vi "Picture to 2-D Color Array.vi"(8 "에러 입력":errorcluster, 10 "입력 클러스터":cluster{"Width":u32, "Height":u32}, 11 "그림":picture) -> (0 "에러 출력":errorcluster, 3 "색 배열":cluster{"Red":u8, "Green":u8, "Blue":u8}[][](array[cluster]))   [LabVIEW 2010]
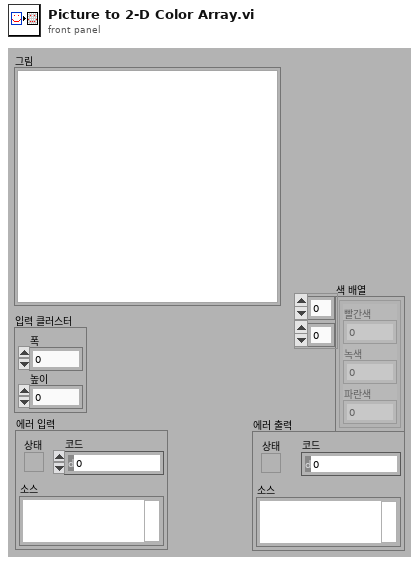
[diagram p1: front panel]
types:
  T1 = cluster{"left":i16, "top":i16, "right":i16, "bottom":i16}
  T2 = typedef "imagedata.ctl" = cluster{"image type":i32, "image depth":i32, "image":u8[], "mask":u8[], "colors":u32[], "Rectangle":cluster{"left":i16, "top":i16, "right":i16, "bottom":i16}}
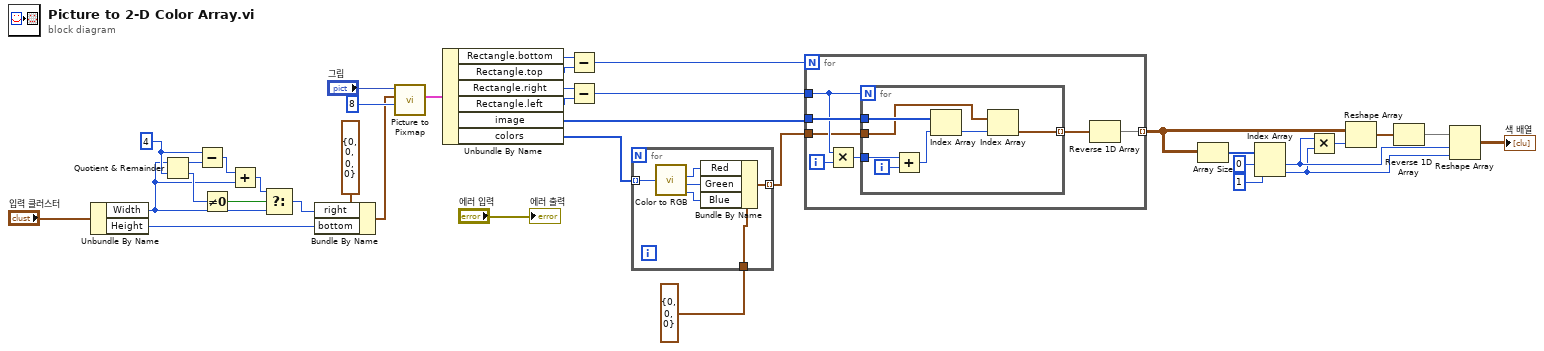
[diagram p0: block diagram]
diagram:
  w21 = 4
  n1 = Unbundle By Name("입력 클러스터") -> ("Width"=w4:u32, "Height"=w25:u32)
  n2 = Quotient & Remainder(x=w4, y=w21) -> (x-y*floor(x/y)=w20:u32, floor(x/y)=w19:u32)
  n3 = Subtract(x=w21, y=w20) -> (x-y=w3:u32)
  n4 = Not Equal To 0?(x=w19) -> (x != 0?=w18:bool)
  n5 = Add(x=w3, y=w4) -> (x+y=w2:u32)
  n6 = Select(t=w2, s=w18, f=w4) -> (s? t:f=w1:u32)
  n7 = Bundle By Name(cluster=T1 {"left"=0, "top"=0, "right"=0, "bottom"=0} ("rect"), "right"=w1, "bottom"=w25) -> (w22:T1)
  n8 = call <vilib>:"Picture to Pixmap.vi"("depth"=8, "rect"=w22, "picture"="그림") -> ("image data"=w26:T2)  [unwired: 7 in, 1 out]
  n9 = Unbundle By Name(w26) -> ("Rectangle.bottom"=w29:i16, "Rectangle.top"=w30:i16, "Rectangle.right"=w32:i16, "Rectangle.left"=w33:i16, "image"=w35:u8[], "colors"=w8:u32[])
  n10 = Subtract(x=w29, y=w30) -> (x-y=w31:i16)
  n11 = Subtract(x=w32, y=w33) -> (x-y=w34:i16)
  n12 = for {
    tunnel: w8 -> [w42] mode=indexing
    tunnel: cluster{"Red":u8, "Green":u8, "Blue":u8} {"Red"=0, "Green"=0, "Blue"=0} ("Cluster") -> [w41]
    tunnel: [w37] -> w6 mode=indexing
    n13 = call <vilib>:"Color to RGB.vi"("Color"=w42) -> ("R"=w39:u8, "G"=w40:u8, "B"=w38:u8)  [unwired: 1 out]
    n14 = Bundle By Name(cluster=w41, "Red"=w39, "Green"=w40, "Blue"=w38) -> (w37:cluster{"Red":u8, "Green":u8, "Blue":u8})
  }
  n15 = for {
    N: w31 -> [_]
    tunnel: w6 -> [w46]
    tunnel: w34 -> [w47]
    tunnel: w35 -> [w49]
    tunnel: [w43] -> w13 mode=indexing
    i -> [w48]
    n16 = Multiply(x=w47, y=w48) -> (x*y=w45:i32)
    n17 = for {
      N: w47 -> [_]
      tunnel: w49 -> [w56]
      tunnel: w46 -> [w51]
      tunnel: w45 -> [w55]
      tunnel: [w50] -> w44 mode=indexing
      i -> [w54]
      n18 = Add(x=w55, y=w54) -> (x+y=w53:i32)
      n19 = Index Array(array=w56, index=w53) -> (element=w52:u8)
      n20 = Index Array(array=w51, index=w52) -> (element=w50:cluster{"Red":u8, "Green":u8, "Blue":u8})
    }
    n21 = Reverse 1D Array(array=w44) -> (reversed array=w43:cluster{"Red":u8, "Green":u8, "Blue":u8}[])
  }
  n22 = Array Size(array=w13) -> (size(s)=w17:i32[])
  n23 = Index Array(array=w17, index #1=0 ("index"), index #2=1 ("index")) -> (element #1=w10:i32, element #2=w9:i32)
  n24 = Multiply(x=w10, y=w9) -> (x*y=w14:i32)
  n25 = Reshape Array(w13, w14) -> (w12:cluster{"Red":u8, "Green":u8, "Blue":u8}[])
  n26 = Reverse 1D Array(array=w12) -> (reversed array=w11:cluster{"Red":u8, "Green":u8, "Blue":u8}[])
  n27 = Reshape Array(w11, w10, w9) -> (→"색 배열":cluster{"Red":u8, "Green":u8, "Blue":u8}[][])
  "에러 출력" <- "에러 입력"
